vi "motor reset.vi"(8 "error in (no error)":errorcluster, 11 "Handle In":i32) -> (0 "error out":errorcluster, 3 "Handle Out":i32)   [LabVIEW 2013]
uses:
  motor constants.ctl
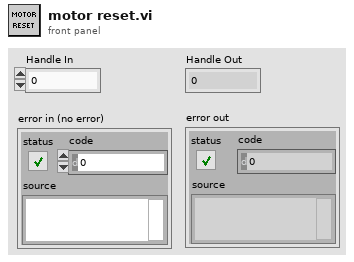
[diagram p1: front panel]
types:
  T1 = typedef "motor constants.ctl" = u16
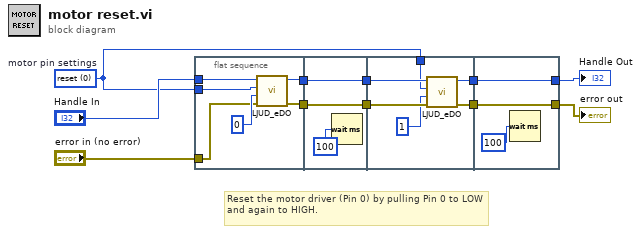
[diagram p0: block diagram]
diagram:
  w3 = T1 0 items=["reset"=0, "error state"=1, "enable"=4, "direction"=5, "step"=6, "end switch"=7]  # motor pin settings
  # "Reset the motor driver (Pin 0) by pulling Pin 0 to LOW and again to HIGH."
  n1 = flat-sequence {
    tunnel: [w15] -> w11
    tunnel: [w16] -> w10
    tunnel: "error in (no error)" -> [w14]
    tunnel: "Handle In" -> [w13]
    tunnel: w3 -> [w12]
    tunnel: [w20] -> w9
    tunnel: w11 -> [w19]
    tunnel: [w19] -> w8
    tunnel: w10 -> [w20]
    tunnel: w9 -> [w26]
    tunnel: [w23] -> w7
    tunnel: w8 -> [w25]
    tunnel: [w24] -> w6
    tunnel: w3 -> [w21]
    tunnel: [w29] -> w2
    tunnel: w7 -> [w29]
    tunnel: [w28] -> w1
    tunnel: w6 -> [w28]
    frame #0 {
      n2 = call <vilib>:"LJUD_eDO.vi"("error in"=w14, "State"=0, "Channel"=w12, "Handle In"=w13) -> ("error out"=w16:errorcluster, "Handle Out"=w15:i32)  [unwired: 6 in]
    }
    frame #1 {
      n3 = Wait (ms)(milliseconds to wait=100) -> ()  [unwired: 1 out]
    }
    frame #2 {
      n4 = call <vilib>:"LJUD_eDO.vi"("error in"=w26, "State"=1, "Channel"=w21, "Handle In"=w25) -> ("error out"=w23:errorcluster, "Handle Out"=w24:i32)  [unwired: 6 in]
    }
    frame #3 {
      n5 = Wait (ms)(milliseconds to wait=100) -> ()  [unwired: 1 out]
    }
  }
  "Handle Out" <- w1
  "error out" <- w2
